vi "main_ctrl.vi"(8 "error in":errorcluster) -> (0 "error out":errorcluster caption="Error")   [LabVIEW 2013]
uses:
  <vilib>/Rock Robotics/WPI/DriverStation/WPI_DriverStationRobotMode2.ctl
  typedefs/fg_typedef.ctl
  typedefs/vision enable.ctl
  typedefs/vision data.ctl
  typedefs/subStates.ctl
  typedefs/singleUseSubstate.ctl
  <vilib>/Rock Robotics/WPI/Solenoid/WPI_SolenoidValue.ctl
  <vilib>/Rock Robotics/WPI/Compressor/WPI_CompressorGetSetRefNum.vi
  <vilib>/Rock Robotics/WPI/RobotDrive/WPI_RobotDriveGetSetRefNum.vi
  <vilib>/Rock Robotics/WPI/Solenoid/WPI_SolenoidSetEnum.vi
  <vilib>/Rock Robotics/WPI/RobotDrive/WPI_RobotDriveArcadeDrive_Standard(NoSaturation).vi
panel:
  out "Robot Mode":T1
  out "Vision SPI":u32
  out "Vision IPS":dbl
  out "Main IPS":dbl
  out "Main SPI":u32
  # "MAIN CONTROL"
  # "holds robot control code - dual parallel state machine"
  # "SPI: milliseconds per iteration\nIPS: iterations per second"
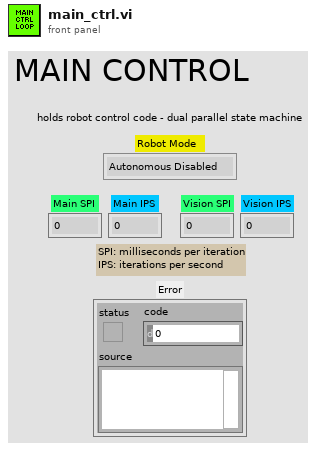
[diagram p1: front panel]
types:
  T1 = typedef "WPI_DriverStationRobotMode2.ctl" = enum16{"Autonomous Disabled", "Autonomous Enabled", "Teleop Disabled", "Teleop Enabled", "Timeout", "Finish", "Test Disabled", "Test Enabled"}
  T2 = typedef "vision data.ctl" = cluster{"x":dbl, "y":dbl, "area":dbl, "width":dbl, "height":dbl, "Hot Goal Present?":bool, "distance":dbl}
  T3 = typedef "vision enable.ctl" = enum16{"Enable", "Disable", "Stop"}
  T4 = typedef "fg_typedef.ctl" = enum16{"Get", "Set"}
  T5 = typedef "WPI_RobotDriveDevRef.ctl" = cluster{"DevStatus":errorcluster, "Motors[]":T6[], "Square Inputs":bool, "Max Output":dbl, "Isochronous":bool}
  T6 = typedef "WPI_MotorControlDeviceRef.ctl" = cluster{"DeviceStatus":errorcluster, "Type":enum16{"PWM", "CAN"}, "PWM":cluster{"Digital Module":T7, "PWM Channel":T8, "DeadBand":T9}, "CAN":cluster{"Device Number":u8, "Control Mode":T10, "Semaphore":T11, "Max Vout":dbl}, "Invert":bool, "TransformRef":T12, "InvTransformRef":T12}
  T7 = typedef "FPGA_TypedefDigitalModule.ctl" = enum16{"Digital Module 1", "Digital Module 2"}
  T8 = typedef "FPGA_DIOPWMChannel.ctl" = enum8{"PWM 1", "PWM 2", "PWM 3", "PWM 4", "PWM 5", "PWM 6", "PWM 7", "PWM 8", "PWM 9", "PWM 10", "Invalid"}
  T9 = typedef "WPI_PWMDeadband.ctl" = cluster{"Name":string, "maxPositivePwm":i32, "minPositivePwm":i32, "centerPwm":i32, "maxNegativePwm":i32, "minNegativePwm":i32, "angularRange":u16}
  T10 = typedef "WPI_CANJaguar_ControlMode.ctl" = enum8{"Percent VBus", "Current", "Speed", "Position", "Voltage"}
  T11 = typedef "Semaphore RefNum" = refnum<k1>
  T12 = typedef "WPI_PWMTransform_ConPane.ctl" = refnum<vi>
  T13 = typedef "WPI_SolenoidDevRef.ctl" = cluster{"DevStatus":errorcluster, "Solenoid Module":T14, "Forward Solenoid Channel":T15, "Reverse Solenoid Channel":T15}
  T14 = typedef "FPGA_TypedefSolenoidModule.ctl" = enum16{"Solenoid Module 1", "Solenoid Module 2"}
  T15 = typedef "WPI_SolenoidChannel.ctl" = enum8{"Solenoid 1", "Solenoid 2", "Solenoid 3", "Solenoid 4", "Solenoid 5", "Solenoid 6", "Solenoid 7", "Solenoid 8", "Invalid"}
  T16 = typedef "WPI_CompressorDevRef.ctl" = cluster{"DevStatus":errorcluster, "DigitalInputDevRef":T17, "RelayDevRef":T19}
  T17 = typedef "WPI_DigitalInputDevRef.ctl" = cluster{"DevStatus":errorcluster, "DIO Channel":T18, "Digital Module":T7}
  T18 = typedef "FPGA_DIOChannel.ctl" = enum8{"DIO 1", "DIO 2", "DIO 3", "DIO 4", "DIO 5", "DIO 6", "DIO 7", "DIO 8", "DIO 9", "DIO 10", "DIO 11", "DIO 12", "DIO 13", "DIO 14", "Invalid"}
  T19 = typedef "WPI_RelayDevRef.ctl" = cluster{"DevStatus":errorcluster, "Relay Channel":T20, "Digital Module":T7, "Relay Direction":T21}
  T20 = typedef "FPGA_DIORelayChannel.ctl" = enum8{"Relay 1", "Relay 2", "Relay 3", "Relay 4", "Relay 5", "Relay 6", "Relay 7", "Relay 8", "Invalid"}
  T21 = typedef "WPI_RelayDirection.ctl" = enum16{"Both directions", "Forward only", "Reverse only"}
  T22 = typedef "WPI_CameraDevRef.ctl" = cluster{"Camera Address":string, "CameraStatus":errorcluster, "Acquire Image Notifier":refnum<notifier>}
  T23 = typedef "IMAQ Image.ctl" = refnum<image>
  T24 = typedef "WPI_SolenoidValue.ctl" = enum16{"Off", "On", "Forward", "Reverse"}
  T25 = typedef "singleUseSubstate.ctl" = enum16{"null", "wait", "shift high", "shift low"}
  T26 = typedef "WPI_DriverStationDerivedRobotMode.ctl" = enum16{"Init", "Execute", "Stop"}
  T27 = typedef "subStates.ctl" = enum16{"null", "wait", "driver control", "auto", "manual override", "hold position", "rotate", "pickup", "pass", "load", "goto shoot", "shoot", "end"}
  T28 = typedef "Loop 2 Datatype.ctl" = cluster{"State":T27, "Waiting Loop":i32, "State to Wait For":i32, "Loop ID":i32, "Exit Value":i32, "Joystick Y":dbl, "Tune Speed":dbl}
  T29 = typedef "Loop 1 Datatype.ctl" = cluster{"State":T27, "Waiting Loop":i32, "State to Wait For":i32, "Loop ID":i32, "Exit Value":i32}
  T30 = typedef "Loop 3 Datatype.ctl" = cluster{"State":T27, "Waiting Loop":i32, "State to Wait For":i32, "Loop ID":i32, "Exit Value":i32, "Joystick Y":dbl, "Joystick Z":dbl}
  T31 = typedef "Loop 0 Datatype.ctl" = cluster{"State":T27, "Waiting Loop":i32, "State to Wait For":i32, "Loop ID":i32, "Exit Value":i32, "X Axis":dbl, "Y Axis":dbl, "Z Axis":dbl}
  T32 = typedef "Loop 4 Datatype.ctl" = cluster{"State":T27, "Waiting Loop":i32, "State to Wait For":i32, "Loop ID":i32, "Exit Value":i32}
  T33 = cluster{"Vision mSPI":u32, "Main mSPI":u32, "Dash mSPI":u32}
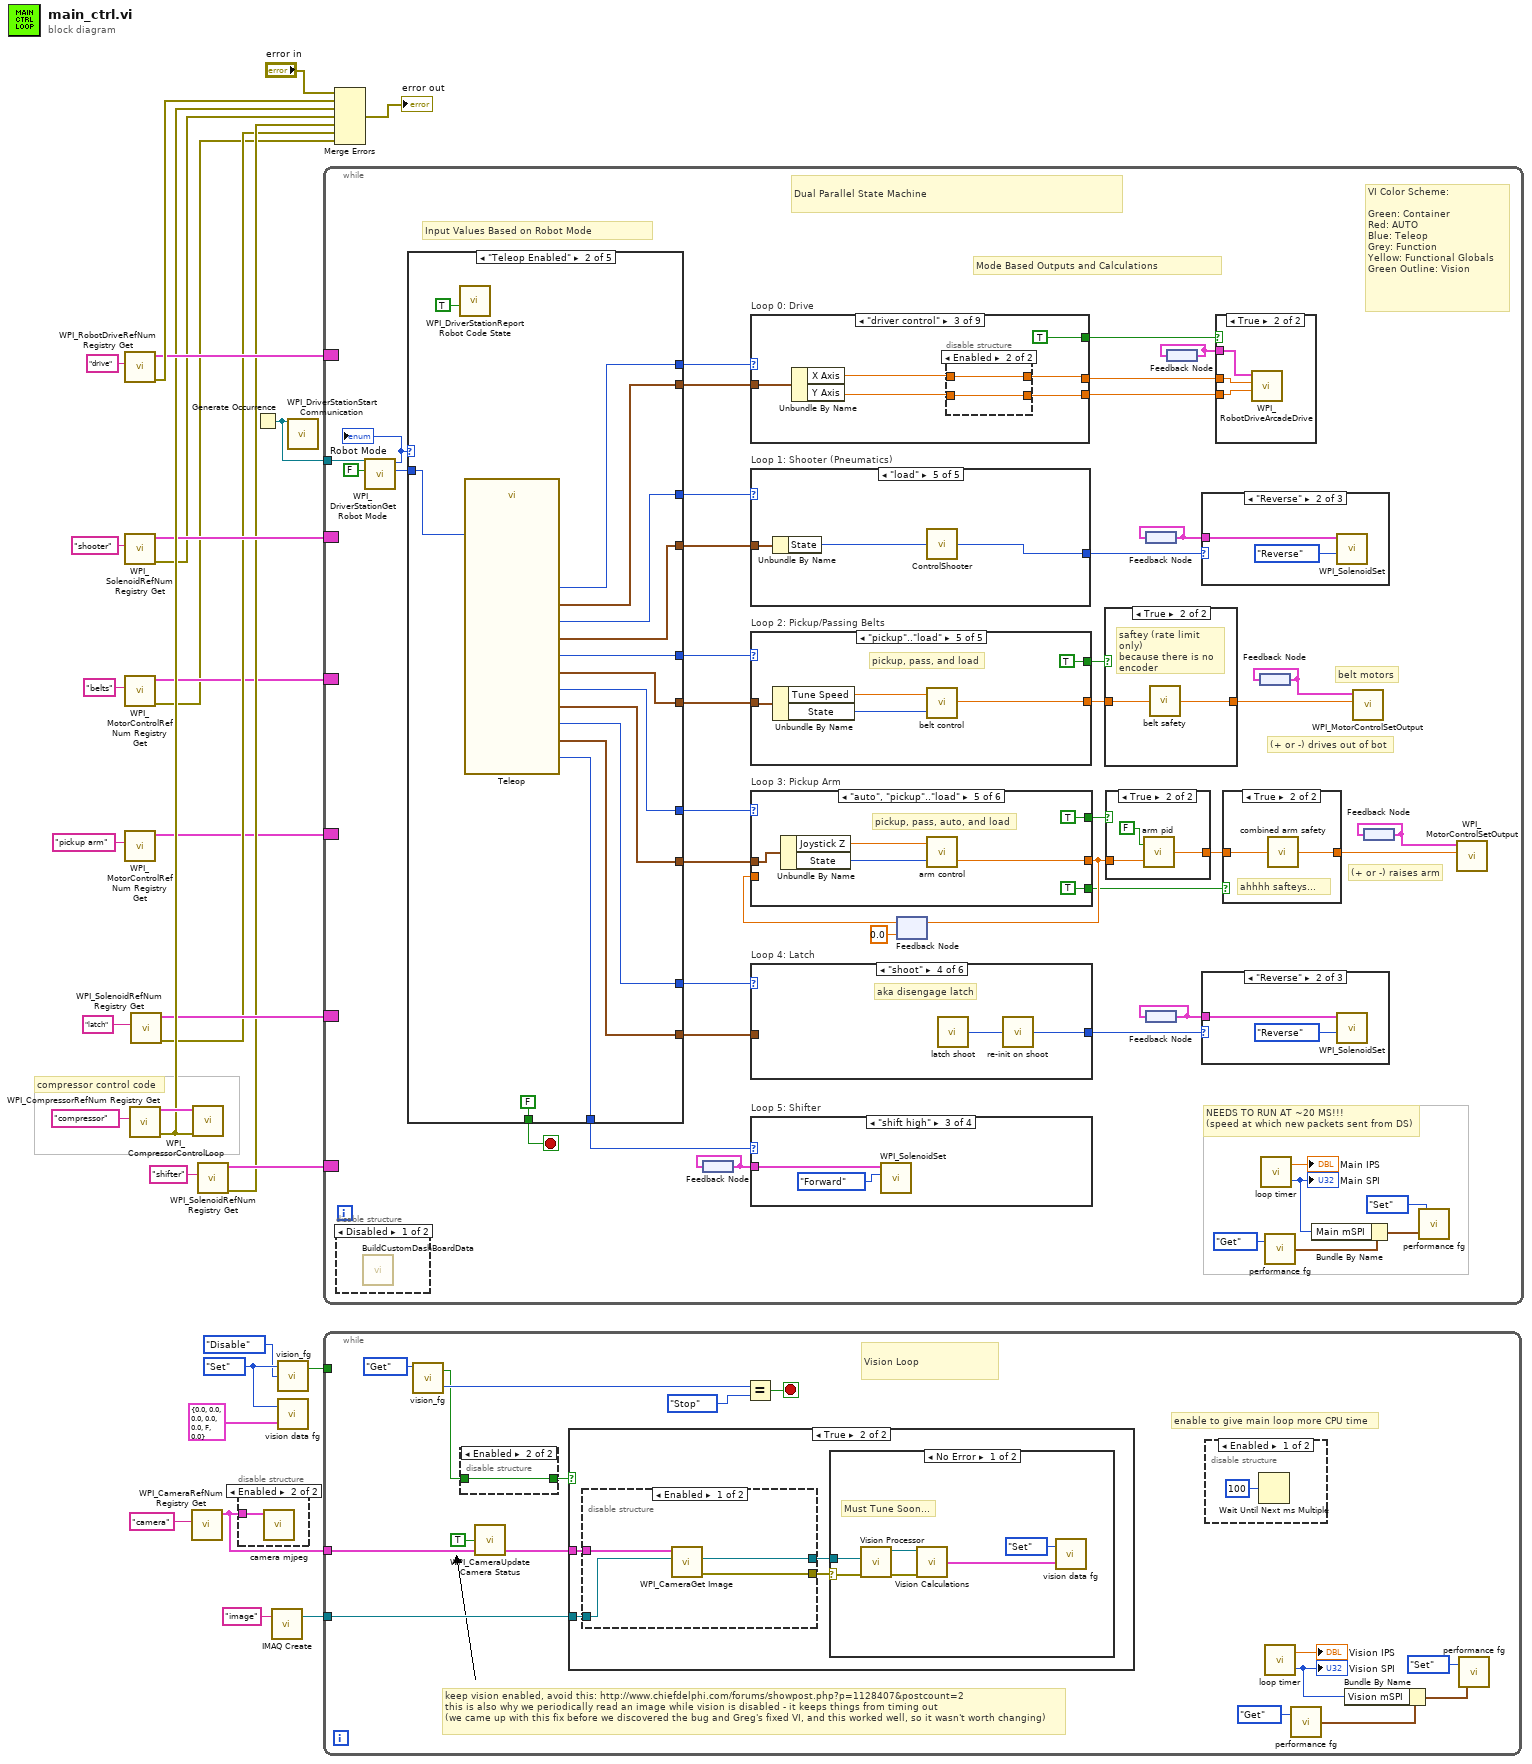
[diagram p0: block diagram]
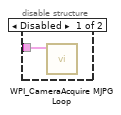
[diagram p2: hidden frame]
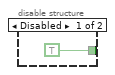
[diagram p3: hidden frame]
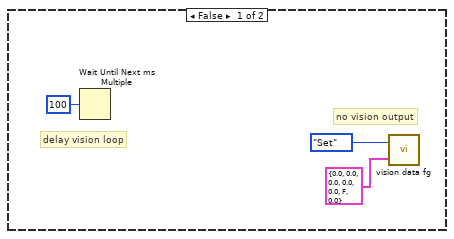
[diagram p5: hidden frame]
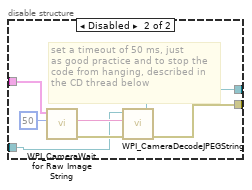
[diagram p7: hidden frame]
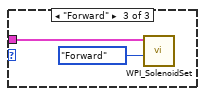
[diagram p12: hidden frame]
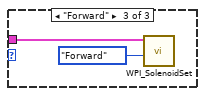
[diagram p14: hidden frame]
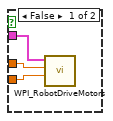
[diagram p16: hidden frame]
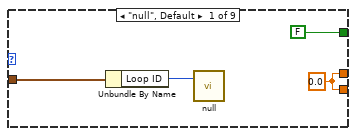
[diagram p17: hidden frame]
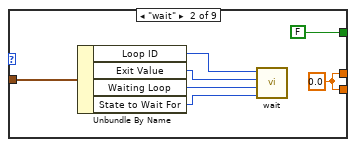
[diagram p18: hidden frame]
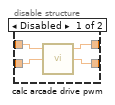
[diagram p19: hidden frame]
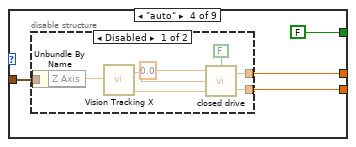
[diagram p20: hidden frame]
diagram:
  w19 = fg_typedef."Set" ("Enum")
  # "compressor control code"
  n1 = call <vilib>:"WPI_RobotDriveRefNum Registry Get.vi"("refnum name"="drive") -> ("error out"=w28:errorcluster, "RobotDriveDevRef"=w26:T5)  [unwired: 9 in]
  n2 = call <vilib>:"WPI_SolenoidRefNum Registry Get.vi"("refnum name"="shooter") -> ("error out"=w7:errorcluster, "SolenoidDevRef"=w11:T13)  [unwired: 9 in]
  n3 = call <vilib>:"WPI_MotorControlRefNum Registry Get.vi"("refnum name"="belts") -> ("error out"=w3:errorcluster, "MotorControlDevRef"=w5:T6)  [unwired: 9 in]
  n4 = call <vilib>:"WPI_MotorControlRefNum Registry Get.vi"("refnum name"="pickup arm") -> ("MotorControlDevRef"=w1:T6)  [unwired: 9 in, 1 out]
  n5 = call <vilib>:"WPI_CompressorRefNum Registry Get.vi"("refnum name"="compressor") -> ("error out"=w22:errorcluster, "CompressorDevRef"=w25:T16)  [unwired: 9 in]
  n6 = call <vilib>:"WPI_SolenoidRefNum Registry Get.vi"("refnum name"="latch") -> ("error out"=w6:errorcluster, "SolenoidDevRef"=w9:T13)  [unwired: 9 in]
  n7 = call <vilib>:"WPI_CameraRefNum Registry Get.vi"("refnum name"="camera") -> ("CameraDevRef"=w16:T22)  [unwired: 9 in, 1 out]
  n8 = call <vilib>:"WPI_CompressorControlLoop.vi"("error in (no error)"=w22, "CompressorDevRef"=w25) -> ()  [unwired: 10 in]
  n9 = call <vilib>:"WPI_SolenoidRefNum Registry Get.vi"("refnum name"="shifter") -> ("error out"=w8:errorcluster, "SolenoidDevRef"=w24:T13)  [unwired: 9 in]
  n10 = disable-structure shown="Enabled" {
    disable-tunnel: w16 -> [w32 w33]
    frame Disabled {
      n11 = call <vilib>:"WPI_CameraAcquire MJPG Loop.vi"("CameraDevRef"=w32) -> ()  [unwired: 11 in]
    }
    frame Enabled {
      n12 = call "camera mjpeg.vi"("CameraDevRef"=w33) -> ()  [unwired: 11 in]
    }
  }
  n13 = Generate Occurrence() -> (w14:refnum<k4>)
  n14 = call "IMAQ Create"("Image Name"="image") -> ("New Image"=w21:T23)  [unwired: 4 in, 1 out]
  n15 = call "vision_fg.vi"("Action"=vision_enable."Disable", "Menu"=w19) -> ("Enabled?"=w20:bool)  [unwired: 1 in, 1 out]
  n16 = call "vision data fg.vi"("Input"=T2 {"x"=0.0, "y"=0.0, "area"=0.0, "width"=0.0, "height"=0.0, "Hot Goal Present?"=FALSE, "distance"=0.0} ("Cluster"), "Menu"=w19) -> ()  [unwired: 1 out]
  n17 = call <vilib>:"WPI_DriverStationStart Communication.vi"("occurrence"=w14) -> ()  [unwired: 11 in]
  n18 = while {
    tunnel: w14 -> [w52]
    border: w26 -> [_]
    border: w24 -> [_]
    border: w11 -> [_]
    border: w9 -> [_]
    border: w5 -> [_]
    border: w1 -> [_]
    stop <- w73 stop-if-true
    # "(+ or -) raises arm"
    # "(+ or -) drives out of bot"
    # "belt motors"
    # "VI Color Scheme:\n\nGreen: Container\nRed: AUTO\nBlue: Teleop\nGrey: Function\nYellow: Functional Globals\nGreen Outline: Vision"
    # "Input Values Based on Robot Mode"
    # "Mode Based Outputs and Calculations"
    # "NEEDS TO RUN AT ~20 MS!!!\n(speed at which new packets sent from DS)"
    # "Dual Parallel State Machine"
    n19 = disable-structure shown="Disabled" {
      frame Disabled {
        n20 = call "BuildCustomDashBoardData.vi"() -> ()  [unwired: 12 in]
      }
      frame Enabled {
      }
    }
    n21 = call <vilib>:"WPI_DriverStationGet Robot Mode.vi"("Finish"=FALSE, "DS Occurrence"=w52) -> ("Call Context"=w51:T26, "Robot Mode"=w50:T1)  [unwired: 8 out]
    "Robot Mode" <- w50
    n22 = case shown="\"Teleop Enabled\"" w50 {
      tunnel: [w261 w278 w280 w286 w292] -> w54
      tunnel: w51 -> [w252 w274 _ _ _]
      tunnel: [w259 w277 w280 w286 w292] -> w75
      tunnel: [w253 w275 singleUseSubstate."null" ("SubState 5") singleUseSubstate."null" ("SubState 5") singleUseSubstate."null" ("SubState 5")] -> w74
      tunnel: [FALSE FALSE FALSE FALSE TRUE] -> w73
      tunnel: [w263 w273 w280 w286 w292] -> w66
      tunnel: [w262 w272 _ _ _] -> w67
      tunnel: [w260 w271 _ _ _] -> w65
      tunnel: [w258 w270 _ _ _] -> w64
      tunnel: [w256 w269 _ _ _] -> w62
      tunnel: [w254 w268 _ _ _] -> w61
      tunnel: [w255 w267 w280 w286 w292] -> w60
      tunnel: [w257 w266 w280 w286 w292] -> w59
      frame "Autonomous Enabled" {
        n23 = call <vilib>:"WPI_DriverStationReport Robot Code State.vi"("Autonomous"=TRUE) -> ()  [unwired: 10 in, 1 out]
        n24 = call "Autonomous.vi"("Call Context"=w252) -> ("SubState 2"=w259:T27, "Loop 2 Data"=w258:T28, "SubState 1"=w261:T27, "Loop 1 Data"=w260:T29, "Loop 3 Data"=w256:T30, "SubState 0"=w263:T27, "SubState 3"=w257:T27, "Loop 0 Data"=w262:T31, "Loop 4 Data"=w254:T32, "SubState 4"=w255:T27, "SubState 5"=w253:T25)
      }
      frame "Teleop Enabled" {
        n25 = call <vilib>:"WPI_DriverStationReport Robot Code State.vi"("TeleOp"=TRUE) -> ()  [unwired: 10 in, 1 out]
        n26 = call "Teleop.vi"("Call Context"=w274) -> ("SubState 3"=w266:T27, "SubState 4"=w267:T27, "SubState 5"=w275:T25, "Loop 3 Data"=w269:T30, "Loop 4 Data"=w268:T32, "SubState 0"=w273:T27, "Loop 1 Data"=w271:T29, "Loop 0 Data"=w272:T31, "SubState 1"=w278:T27, "Loop 2 Data"=w270:T28, "SubState 2"=w277:T27)  [unwired: 8 in]
      }
      frame "Autonomous Disabled", "Teleop Disabled", "Timeout" {
        w280 = subStates."null" ("SubState 0")
        # "set all loops to null"
        # "make sure to disable vision\nwe don't need it here"
        # "robot disabled, timeout"
        n27 = call <vilib>:"WPI_DriverStationReport Robot Code State.vi"("Disabled"=TRUE) -> ()  [unwired: 10 in, 1 out]
        n28 = call "vision_fg.vi"("Action"=vision_enable."Disable", "Menu"=fg_typedef."Set") -> ()  [unwired: 1 in, 2 out]
      }
      frame "Test Disabled", "Test Enabled" {
        w286 = subStates."null" ("SubState 0")
        # "set all loops to null"
        # "make sure to disable vision\nwe don't need it here"
        # "test, unused"
        n29 = call <vilib>:"WPI_DriverStationReport Robot Code State.vi"("Test"=TRUE) -> ()  [unwired: 10 in, 1 out]
        n30 = call "vision_fg.vi"("Action"=vision_enable."Disable", "Menu"=fg_typedef."Set") -> ()  [unwired: 1 in, 2 out]
      }
      frame "Finish" {
        w292 = subStates."end"  # Stop All Loops
        # "stop the while loop"
        # "stop DS comms"
        # "stop vision loop"
        n31 = call <vilib>:"WPI_DriverStationStop Communication.vi"("StopCommunication"=TRUE) -> ()  [unwired: 10 in, 1 out]
        n32 = call "vision_fg.vi"("Action"=vision_enable."Stop", "Menu"=fg_typedef."Set") -> ()  [unwired: 1 in, 2 out]
      }
    }
    n33 = feedback #1() -> (w63:T13)
    n34 = feedback-in #1(w63) -> ()
    n35 = case "Loop 0: Drive" shown="\"driver control\"" w66 {
      tunnel: w67 -> [w103 w107 w117 w124 w141 w148 _ _ w164]
      tunnel: [w101 w105 w113 w126 w138 w150 w153 w158 w160] -> w57
      tunnel: [w101 w105 w112 w125 w137 w149 w152 w158 w159] -> w56
      tunnel: [FALSE FALSE TRUE FALSE FALSE FALSE FALSE FALSE FALSE] -> w58
      frame "null", Default {
        w101 = 0.0 ("X Axis")
        n36 = Unbundle By Name(w103) -> ("Loop ID"=w104:i32)
        n37 = call "null.vi"("This Loop ID"=w104) -> ()  [unwired: 2 in]
      }
      frame "wait" {
        w105 = 0.0 ("X Axis")
        n38 = Unbundle By Name(w107) -> ("Loop ID"=w111:i32, "Exit Value"=w110:i32, "Waiting Loop"=w109:i32, "State to Wait For"=w108:i32)
        n39 = call "wait.vi"("State to wait for"=w108, "Waiting Loop ID"=w109, "time (ms)"=w110, "Current Loop ID"=w111) -> ()  [unwired: 1 out]
      }
      frame "driver control" {
        n40 = Unbundle By Name(w117) -> ("X Axis"=w115:dbl, "Y Axis"=w114:dbl)
        n41 = disable-structure shown="Enabled" {
          disable-tunnel: w115 -> [w121 w123]
          disable-tunnel: w114 -> [w120 w122]
          disable-tunnel: [w119 w123] -> w113
          disable-tunnel: [w118 w122] -> w112
          frame Disabled {
            n42 = call "calc arcade drive pwm.vi"("Y axis value"=w120, "X axis value"=w121) -> ("Right Speed"=w118:dbl, "Left Speed"=w119:dbl)  [unwired: 1 in, 1 out]
          }
          frame Enabled {
          }
        }
      }
      frame "auto" {
        n43 = disable-structure shown="Disabled" {
          disable-tunnel: [w135 _] -> w126
          disable-tunnel: [w134 _] -> w125
          disable-tunnel: w124 -> [w130 _]
          frame Disabled {
            n44 = Unbundle By Name(w130) -> ("Z Axis"=w128:dbl)
            n45 = call "Vision Tracking X.vi"("Tweak"=w128) -> ("right speed"=w129:dbl, "left speed"=w132:dbl)
            n46 = call "closed drive.vi"("Acrade Drive?"=FALSE, "Y axis value (Left)"=w132, "X axis value (Right)"=w129, "Threshold (.4)"=0.0 ("Threshold")) -> ("right"=w134:dbl, "left"=w135:dbl)
          }
          frame Enabled {
            # "rotates toward target"
            # "not in use this year"
          }
        }
      }
      frame "hold position" {
        n47 = Unbundle By Name(w141) -> ("X Axis"=w140:dbl, "Y Axis"=w139:dbl)
        n48 = call "closed drive.vi"("Acrade Drive?"=TRUE, "Y axis value (Left)"=w139, "X axis value (Right)"=w140) -> ("right"=w137:dbl, "left"=w138:dbl)  [unwired: 1 in]
      }
      frame "rotate" {
        # "use these to carry actual information because this is\nfor autonomous only so there will not be joystick input"
        n49 = Unbundle By Name(w148) -> ("X Axis"=w147:dbl, "Y Axis"=w146:dbl)
        n50 = call "rotate.vi"("Angle"=w147, "Rate"=w146) -> ("finished?"=w143:bool, "left speed"=w150:dbl, "right speed"=w149:dbl)
        n51 = call "states FG.vi"("exit in"=w143, "menu (get)"=enum16{"set", "get"}."set", "Loop ID"=0) -> ()  [unwired: 5 in, 4 out]
      }
      frame "goto shoot" {
        # "consider implimenting closed hold with drive"
        n52 = call "vision data fg.vi"("Menu"=fg_typedef."Get") -> ("Output"=w154:T2)  [unwired: 1 in]
        n53 = call "goto location.vi"("Image Data"=w154) -> ("left speed"=w153:dbl, "right speed"=w152:dbl)
      }
      frame "end" {
        w158 = 0.0 ("X Axis")
      }
      frame "manual override" {
        n54 = Unbundle By Name(w164) -> ("X Axis"=w163:dbl, "Y Axis"=w162:dbl)
        n55 = expression code="x/2"(w163) -> (w160:dbl)
        n56 = expression code="x/2"(w162) -> (w159:dbl)
      }
    }
    n57 = case "Loop 1: Shooter (Pneumatics)" shown="\"load\"" w54 {
      tunnel: w65 -> [w238 w241 _ _ w250]
      tunnel: [WPI_SolenoidValue."Off" ("Value") WPI_SolenoidValue."Off" ("Value") WPI_SolenoidValue."Off" ("Value") WPI_SolenoidValue."Off" ("Value") w248] -> w49
      frame "null", Default {
        n58 = Unbundle By Name(w238) -> ("Loop ID"=w239:i32)
        n59 = call "null.vi"("This Loop ID"=w239) -> ()  [unwired: 2 in]
      }
      frame "wait" {
        n60 = Unbundle By Name(w241) -> ("Loop ID"=w245:i32, "Exit Value"=w244:i32, "Waiting Loop"=w243:i32, "State to Wait For"=w242:i32)
        n61 = call "wait.vi"("State to wait for"=w242, "Waiting Loop ID"=w243, "time (ms)"=w244, "Current Loop ID"=w245) -> ()  [unwired: 1 out]
      }
      frame "driver control" {
      }
      frame "manual override" {
      }
      frame "load" {
        n62 = Unbundle By Name(w250) -> ("State"=w249:T27)
        n63 = call "ControlShooter.vi"("State"=w249) -> ("To Shooter\nSolenoid Loop"=w248:T24)
      }
    }
    n64 = case "Loop 2: Pickup/Passing Belts" shown="\"pickup\"..\"load\"" w75 {
      tunnel: w64 -> [w217 w220 w227 w231 w236]
      tunnel: [0.0 ("output") 0.0 ("output") w226 w229 w233] -> w35
      tunnel: [FALSE FALSE TRUE FALSE TRUE] -> w36
      frame "null", Default {
        n65 = Unbundle By Name(w217) -> ("Loop ID"=w216:i32)
        n66 = call "null.vi"("This Loop ID"=w216) -> ()  [unwired: 2 in]
      }
      frame "wait" {
        n67 = Unbundle By Name(w220) -> ("Loop ID"=w224:i32, "Exit Value"=w223:i32, "Waiting Loop"=w222:i32, "State to Wait For"=w221:i32)
        n68 = call "wait.vi"("State to wait for"=w221, "Waiting Loop ID"=w222, "time (ms)"=w223, "Current Loop ID"=w224) -> ()  [unwired: 1 out]
      }
      frame "driver control" {
        n69 = Unbundle By Name(w227) -> ("Joystick Y"=w226:dbl)
      }
      frame "manual override" {
        n70 = Unbundle By Name(w231) -> ("Joystick Y"=w230:dbl)
        n71 = expression code="x/2"(w230) -> (w229:dbl)
      }
      frame "pickup".."load" {
        # "pickup, pass, and load"
        n72 = Unbundle By Name(w236) -> ("Tune Speed"=w235:dbl, "State"=w234:T27)
        n73 = call "belt control.vi"("State"=w234, "Joystick Z"=w235) -> ("output"=w233:dbl)
      }
    }
    n74 = case "Loop 4: Latch" shown="\"shoot\"" w60 {
      tunnel: w61 -> [w167 w169 _ _ _ _]
      tunnel: [WPI_SolenoidValue."Off" ("Value") WPI_SolenoidValue."Off" ("Value") WPI_SolenoidValue."Off" ("Value") w175 WPI_SolenoidValue."Forward" ("Value") WPI_SolenoidValue."Reverse" ("Value")] -> w46
      frame "null", Default {
        n75 = Unbundle By Name(w167) -> ("Loop ID"=w166:i32)
        n76 = call "null.vi"("This Loop ID"=w166) -> ()  [unwired: 2 in]
      }
      frame "wait" {
        n77 = Unbundle By Name(w169) -> ("Loop ID"=w173:i32, "Exit Value"=w172:i32, "Waiting Loop"=w171:i32, "State to Wait For"=w170:i32)
        n78 = call "wait.vi"("State to wait for"=w170, "Waiting Loop ID"=w171, "time (ms)"=w172, "Current Loop ID"=w173) -> ()  [unwired: 1 out]
      }
      frame "driver control" {
      }
      frame "shoot" {
        # "aka disengage latch"
        n79 = call "latch shoot.vi"() -> ("Latch"=w176:T24)
        n80 = call "re-init on shoot.vi"("Relay Value"=w176) -> ("Value"=w175:T24)
      }
      frame "auto" {
        # "aka engage"
      }
      frame "manual override" {
        # "unsafely shoot"
      }
    }
    n81 = case "Loop 5: Shifter" shown="\"shift high\"" w74 {
      tunnel: w63 -> [_ _ w211 w212]
      frame "null", Default {
      }
      frame "wait" {
      }
      frame "shift high" {
        n82 = call-poly <vilib>:"WPI_SolenoidSet.vi"("Value"=WPI_SolenoidValue."Forward", "SolenoidDevRef"=w211) -> ()  [unwired: 8 in, 2 out]
      }
      frame "shift low" {
        n83 = call-poly <vilib>:"WPI_SolenoidSet.vi"("Value"=WPI_SolenoidValue."Reverse", "SolenoidDevRef"=w212) -> ()  [unwired: 8 in, 2 out]
      }
    }
    n84 = feedback #2(0.0 ("output")) -> (w41:dbl)
    n85 = case "Loop 3: Pickup Arm" shown="\"auto\", \"pickup\"..\"load\"" w59 {
      tunnel: w62 -> [w183 w187 w194 w200 w206 _]
      tunnel: [FALSE FALSE FALSE FALSE TRUE TRUE] -> w43
      tunnel: [0.0 ("output") 0.0 ("output") w193 w198 w202 w208] -> w42
      tunnel: w41 -> [_ _ _ _ _ w208]
      tunnel: [TRUE TRUE TRUE FALSE TRUE TRUE] -> w39
      frame "null", Default {
        n86 = Unbundle By Name(w183) -> ("Loop ID"=w182:i32)
        n87 = call "null.vi"("This Loop ID"=w182) -> ()  [unwired: 2 in]
      }
      frame "wait" {
        n88 = Unbundle By Name(w187) -> ("Loop ID"=w191:i32, "Exit Value"=w190:i32, "Waiting Loop"=w189:i32, "State to Wait For"=w188:i32)
        n89 = call "wait.vi"("State to wait for"=w188, "Waiting Loop ID"=w189, "time (ms)"=w190, "Current Loop ID"=w191) -> ()  [unwired: 1 out]
      }
      frame "driver control" {
        n90 = Unbundle By Name(w194) -> ("Joystick Y"=w193:dbl)
      }
      frame "manual override" {
        n91 = Unbundle By Name(w200) -> ("Joystick Y"=w199:dbl)
        n92 = expression code="x/2"(w199) -> (w198:dbl)
      }
      frame "auto", "pickup".."load" {
        # "pickup, pass, auto, and load"
        n93 = Unbundle By Name(w206) -> ("Joystick Z"=w204:dbl, "State"=w203:T27)
        n94 = call "arm control.vi"("State"=w203, "Z Axis (Tuning)"=w204) -> ("setpoint"=w202:dbl)
      }
      frame "hold position" {
      }
    }
    n95 = feedback-in #2(w42) -> ()
    n96 = case shown="True" w36 {
      tunnel: w35 -> [w77 w79]
      tunnel: [w77 w78] -> w34
      frame False {
        # "no saftey"
      }
      frame True {
        # "saftey (rate limit only)\nbecause there is no \nencoder"
        n97 = call "belt safety.vi"("Input"=w79) -> ("Safe Output"=w78:dbl)
      }
    }
    n98 = case shown="True" w43 {
      tunnel: w42 -> [w83 w86]
      tunnel: [w83 w85] -> w38
      frame False {
        # "open loop"
      }
      frame True {
        n99 = call "arm pid.vi"("Setpoint"=w86, "Autotune?"=FALSE) -> ("Output"=w85:dbl)
      }
    }
    n100 = feedback #3() -> (w48:T13)
    n101 = feedback-in #3(w48) -> ()
    n102 = feedback #4() -> (w47:T13)
    n103 = feedback-in #4(w47) -> ()
    n104 = feedback #5() -> (w55:T5)
    n105 = feedback-in #5(w55) -> ()
    n106 = case shown="\"Reverse\"" w49 {
      tunnel: w48 -> [_ w91 w93]
      frame "Off", Default {
      }
      frame "Reverse" {
        n107 = call-poly <vilib>:"WPI_SolenoidSet.vi"("Value"=WPI_SolenoidValue."Reverse", "SolenoidDevRef"=w91) -> ()  [unwired: 8 in, 2 out]
      }
      frame "Forward" {
        n108 = call-poly <vilib>:"WPI_SolenoidSet.vi"("Value"=WPI_SolenoidValue."Forward", "SolenoidDevRef"=w93) -> ()  [unwired: 8 in, 2 out]
      }
    }
    n109 = case shown="\"Reverse\"" w46 {
      tunnel: w47 -> [_ w87 w89]
      frame "Off", Default {
      }
      frame "Reverse" {
        n110 = call-poly <vilib>:"WPI_SolenoidSet.vi"("Value"=WPI_SolenoidValue."Reverse", "SolenoidDevRef"=w87) -> ()  [unwired: 8 in, 2 out]
      }
      frame "Forward" {
        n111 = call-poly <vilib>:"WPI_SolenoidSet.vi"("Value"=WPI_SolenoidValue."Forward", "SolenoidDevRef"=w89) -> ()  [unwired: 8 in, 2 out]
      }
    }
    n112 = case shown="True" w58 {
      tunnel: w57 -> [w96 w100]
      tunnel: w56 -> [w95 w99]
      tunnel: w55 -> [w97 w98]
      frame False {
        n113 = call <vilib>:"WPI_RobotDriveMotors.vi"("RightSpeed"=w95, "LeftSpeed"=w96, "RobotDriveDevRef"=w97) -> ()  [unwired: 6 in, 3 out]
      }
      frame True {
        n114 = call-poly <vilib>:"WPI_RobotDriveArcadeDrive.vi"("Y axis value"=w99, "X axis value"=w100, "RobotDriveDevRef"=w98) -> ()  [unwired: 6 in, 3 out]
      }
    }
    n115 = case shown="True" w39 {
      tunnel: w38 -> [w80 w82]
      tunnel: [w80 w81] -> w37
      frame False {
        # "no saftey???"
      }
      frame True {
        # "ahhhh safteys..."
        n116 = call "combined arm safety.vi"("Input"=w82) -> ("Safe Output"=w81:dbl)
      }
    }
    n117 = feedback #6() -> (w45:T6)
    n118 = feedback-in #6(w45) -> ()
    n119 = call "loop timer.vi"() -> ("IPS"=→"Main IPS":dbl, "SPI"=w72:u32)  [unwired: 1 in]
    "Main SPI" <- w72
    n120 = call "performance fg.vi"("Menu"=fg_typedef."Get") -> ("Output"=w69:T33)  [unwired: 1 in]
    n121 = Bundle By Name(cluster=w69, "Main mSPI"=w72) -> (w68:T33)
    n122 = call <vilib>:"WPI_MotorControlSetOutput.vi"("Output"=w34, "MotorControlDevRef"=w45) -> ()  [unwired: 7 in, 3 out]
    n123 = feedback #7() -> (w44:T6)
    n124 = feedback-in #7(w44) -> ()
    n125 = call "performance fg.vi"("Input"=w68, "Menu"=fg_typedef."Set") -> ()  [unwired: 1 out]
    n126 = call <vilib>:"WPI_MotorControlSetOutput.vi"("Output"=w37, "MotorControlDevRef"=w44) -> ()  [unwired: 7 in, 3 out]
  }
  n127 = while {
    tunnel: w21 -> [w311]
    tunnel: w16 -> [w310]
    tunnel: w20 -> [_]
    stop <- w312 stop-if-true
    # "keep vision enabled, avoid this: http://www.chiefdelphi.com/forums/showpost.php?p=1128407&postcount=2\nthis is also why we periodically read an image while vision is disabled - it keeps things from timing out\n(we came up with this fix before we discovered the bug and Greg's fixed VI, and this worked well, so it wasn't worth changing)"
    # "enable to give main loop more CPU time"
    # "Vision Loop"
    n128 = call "vision_fg.vi"("Menu"=fg_typedef."Get" ("Enum")) -> ("State Out"=w306:T3, "Enabled?"=w297:bool)  [unwired: 2 in]
    n129 = disable-structure shown="Enabled" {
      disable-tunnel: [TRUE w314] -> w298
      disable-tunnel: w297 -> [_ w314]
      frame Disabled {
      }
      frame Enabled {
      }
    }
    n130 = call <vilib>:"WPI_CameraUpdate Camera Status.vi"("CameraDevRef In"=w310, "Enable Vision"=TRUE) -> ("CameraDevRef Out"=w309:T22)  [unwired: 3 in]
    n131 = case shown="True" w298 {
      tunnel: w311 -> [_ w322]
      tunnel: w309 -> [_ w321]
      frame False {
        # "no vision output"
        # "delay vision loop"
        n132 = Wait Until Next ms Multiple(millisecond multiple=u32 100) -> ()  [unwired: 1 out]
        n133 = call "vision data fg.vi"("Input"=T2 {"x"=0.0, "y"=0.0, "area"=0.0, "width"=0.0, "height"=0.0, "Hot Goal Present?"=FALSE, "distance"=0.0} ("Cluster"), "Menu"=fg_typedef."Set" ("Enum")) -> ()  [unwired: 1 out]
      }
      frame True {
        n134 = disable-structure shown="Enabled" {
          disable-tunnel: w322 -> [w331 w335]
          disable-tunnel: w321 -> [w332 w337]
          disable-tunnel: [w330 w334] -> w320
          disable-tunnel: [w329 w333] -> w319
          frame Enabled {
            n135 = call <vilib>:"WPI_CameraGet Image.vi"("Image"=w331, "CameraDevRef"=w332) -> ("error out"=w329:errorcluster, "Image Out"=w330:T23)  [unwired: 7 in, 1 out]
          }
          frame Disabled {
            # "set a timeout of 50 ms, just\nas good practice and to stop the \ncode from hanging, described in \nthe CD thread below"
            n136 = call <vilib>:"WPI_CameraWait for Raw Image String.vi"("Timeout in ms (-1)"=50, "CameraDevRef"=w337) -> ("error out"=w339:errorcluster, "String"=w338:string)  [unwired: 3 in, 5 out]
            n137 = call <vilib>:"WPI_CameraDecodeJPEGString.vi"("error in"=w339, "Compressed Image"=w338, "Image In"=w335) -> ("error out"=w333:errorcluster, "Image Out"=w334:T23)  [unwired: 3 out]
          }
        }
        n138 = case shown="No Error" w319 {
          selector: w319 -> [w327 _]
          tunnel: w320 -> [w326 _]
          frame No Error {
            # "Must Tune Soon..."
            n139 = call "Vision Processor.vi"("error in"=w327, "Image In"=w326) -> ("error out"=w324:errorcluster, "Image Out"=w325:T23)  [unwired: 5 in]
            n140 = call "Vision Calculations.vi"("Image In"=w325, "error in"=w324) -> ("Vision Data"=w323:T2)  [unwired: 3 in]
            n141 = call "vision data fg.vi"("Input"=w323, "Menu"=fg_typedef."Set" ("Enum")) -> ()  [unwired: 1 out]
          }
          frame Error {
          }
        }
      }
    }
    n142 = Equal?(x=w306, y=vision_enable."Stop") -> (x = y?=w312:bool)
    n143 = disable-structure shown="Enabled" {
      frame Enabled {
        n144 = Wait Until Next ms Multiple(millisecond multiple=u32 100) -> ()  [unwired: 1 out]
      }
      frame Disabled {
      }
    }
    n145 = call "loop timer.vi"() -> ("IPS"=→"Vision IPS":dbl, "SPI"=w304:u32)  [unwired: 1 in]
    "Vision SPI" <- w304
    n146 = call "performance fg.vi"("Menu"=fg_typedef."Get") -> ("Output"=w302:T33)  [unwired: 1 in]
    n147 = Bundle By Name(cluster=w302, "Vision mSPI"=w304) -> (w301:T33)
    n148 = call "performance fg.vi"("Input"=w301, "Menu"=fg_typedef."Set") -> ()  [unwired: 1 out]
  }
  n149 = Merge Errors("error in", w28, w22, w7, w8, w6, w3) -> (→"error out":errorcluster)
